vi "Save Object Settings.vi"(8 "error in":errorcluster, 10 "Settings":T5={"Paths"=[refnum, refnum, refnum], "Rectangles"=[refnum, refnum], "Funnels"=[refnum, refnum, refnum, refnum, refnum, refnum], "Dots"=[refnum, refnum, refnum, refnum, refnum, refnum, refnum, refnum, refnum]}, 11 "Archivist in":refnum<class "Archivist.lvclass">) -> (0 "error out":errorcluster, 3 "Archivist out":refnum<class "Archivist.lvclass">)   [LabVIEW 2019, in "Archivist.lvclass"]
uses:
  Archivist.lvclass
  Settings/Setting Database/Typedefs/PublicEvents--Setting Database.PathsUpdated.ctl
  Settings/Path Settings/Path Settings.lvclass
  Settings/Setting Database/Typedefs/PublicEvents--Setting Database.RectanglesUpdated.ctl
  Settings/Rectangle Settings/Rectangle Settings.lvclass
  Settings/Setting Database/Typedefs/PublicEvents--Setting Database.FunnelsUpdated.ctl
  Settings/Funnel Settings/Funnel Settings.lvclass
  Settings/Setting Database/Typedefs/PublicEvents--Setting Database.DotsUpdated.ctl
  Settings/Dot Settings/Dot Settings.lvclass
  Settings/Setting Database/Setting Database.lvclass
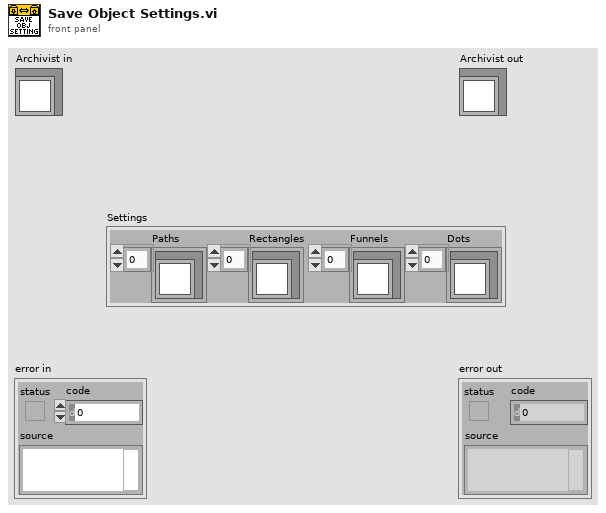
[diagram p1: front panel]
types:
  T1 = typedef "Setting Database.lvclass/PublicEvents--Setting Database.PathsUpdated.ctl" = refnum<class "Path Settings.lvclass">[]
  T2 = typedef "Setting Database.lvclass/PublicEvents--Setting Database.RectanglesUpdated.ctl" = refnum<class "Rectangle Settings.lvclass">[]
  T3 = typedef "Setting Database.lvclass/PublicEvents--Setting Database.FunnelsUpdated.ctl" = refnum<class "Funnel Settings.lvclass">[]
  T4 = typedef "Setting Database.lvclass/PublicEvents--Setting Database.DotsUpdated.ctl" = refnum<class "Dot Settings.lvclass">[]
  T5 = cluster{"Paths":T1, "Rectangles":T2, "Funnels":T3, "Dots":T4}
  T6 = enum16{"open", "replace", "create", "open or create", "replace or create", "replace or create with confirmation"}
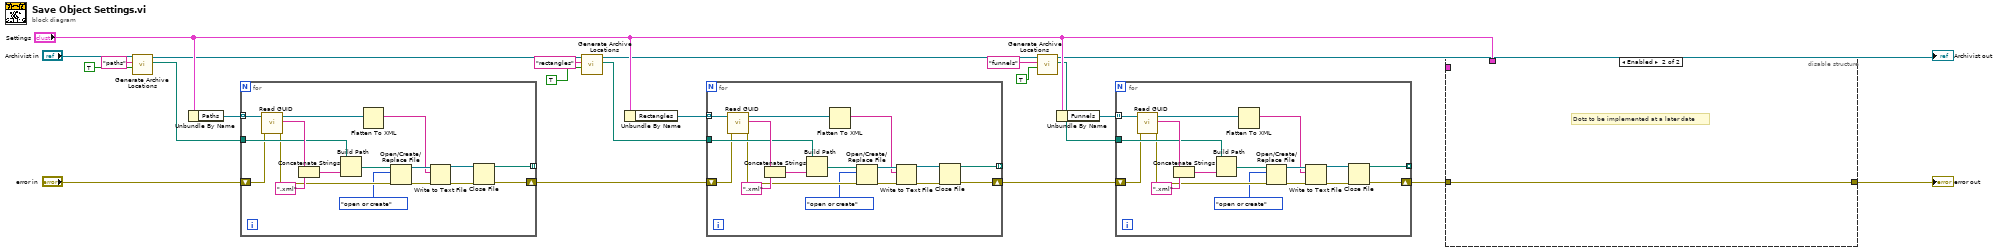
[diagram p0: block diagram]
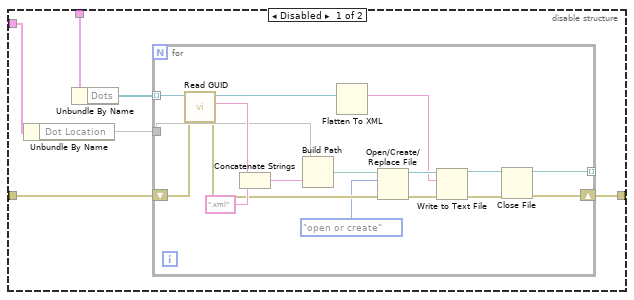
[diagram p2: hidden frame]
diagram:
  n1 = call "Generate Archive Locations.vi"("Archive?"=TRUE, "Key"="paths", "Archivist In"="Archivist in") -> ("Path Out"=w13:path, "Archivist Out"=w10:refnum<class "Archivist.lvclass">)  [unwired: 7 in]
  n2 = Unbundle By Name("Settings") -> ("Paths"=w21:T1)
  n3 = for {
    tunnel: w13 -> [w36]
    tunnel: w21 -> [w39] mode=indexing
    tunnel: [w27] -> _ mode=indexing
    shift-right: [w26] -> w3
    shift-left: "error in" -> [w25]
    n4 = call-dynamic "Read GUID.vi"("error in (no error)"=w25, "ObjectSettings in"=w39) -> ("error out"=w30:errorcluster, "GUID"=w37:string, "ObjectSettings out"=w34:refnum<class "Path Settings.lvclass">)  [unwired: 7 in]
    n5 = Concatenate Strings(w37, ".xml" ("string")) -> (w35:string)
    n6 = Build Path(base path=w36, name or relative path=w35) -> (appended path=w33:path)
    n7 = Flatten To XML(anything=w34) -> (xml string=w24:string)
    n8 = Open/Create/Replace File(file path (use dialog)=w33, error in=w30, operation (0:open)=T6."open or create") -> (refnum out=w32:refnum<file>, error out=w31:errorcluster)  [unwired: 3 in, 1 out]
    n9 = Write to Text File(file (use dialog)=w32, text=w24, error in=w31) -> (refnum out=w28:refnum<file>, error out=w29:errorcluster)  [unwired: 1 in, 1 out]
    n10 = Close File(refnum=w28, error in=w29) -> (path=w27:path, error out=w26:errorcluster)
  }
  n11 = call "Generate Archive Locations.vi"("Archive?"=TRUE, "Key"="rectangles", "Archivist In"=w10) -> ("Path Out"=w9:path, "Archivist Out"=w7:refnum<class "Archivist.lvclass">)  [unwired: 7 in]
  n12 = Unbundle By Name("Settings") -> ("Rectangles"=w20:T2)
  n13 = for {
    tunnel: w9 -> [w53]
    tunnel: w20 -> [w56] mode=indexing
    tunnel: [w44] -> _ mode=indexing
    shift-right: [w43] -> w2
    shift-left: w3 -> [w42]
    n14 = call-dynamic "Read GUID.vi"("error in (no error)"=w42, "ObjectSettings in"=w56) -> ("error out"=w47:errorcluster, "GUID"=w54:string, "ObjectSettings out"=w51:refnum<class "Rectangle Settings.lvclass">)  [unwired: 7 in]
    n15 = Concatenate Strings(w54, ".xml" ("string")) -> (w52:string)
    n16 = Build Path(base path=w53, name or relative path=w52) -> (appended path=w50:path)
    n17 = Flatten To XML(anything=w51) -> (xml string=w41:string)
    n18 = Open/Create/Replace File(file path (use dialog)=w50, error in=w47, operation (0:open)=T6."open or create") -> (refnum out=w49:refnum<file>, error out=w48:errorcluster)  [unwired: 3 in, 1 out]
    n19 = Write to Text File(file (use dialog)=w49, text=w41, error in=w48) -> (refnum out=w45:refnum<file>, error out=w46:errorcluster)  [unwired: 1 in, 1 out]
    n20 = Close File(refnum=w45, error in=w46) -> (path=w44:path, error out=w43:errorcluster)
  }
  n21 = call "Generate Archive Locations.vi"("Archive?"=TRUE, "Key"="funnels", "Archivist In"=w7) -> ("Path Out"=w5:path, "Archivist Out"=→"Archivist out":refnum<class "Archivist.lvclass">)  [unwired: 7 in]
  n22 = Unbundle By Name("Settings") -> ("Funnels"=w19:T3)
  n23 = for {
    tunnel: w5 -> [w70]
    tunnel: w19 -> [w73] mode=indexing
    tunnel: [w61] -> _ mode=indexing
    shift-right: [w60] -> w18
    shift-left: w2 -> [w59]
    n24 = call-dynamic "Read GUID.vi"("error in (no error)"=w59, "ObjectSettings in"=w73) -> ("error out"=w64:errorcluster, "GUID"=w71:string, "ObjectSettings out"=w68:refnum<class "Funnel Settings.lvclass">)  [unwired: 7 in]
    n25 = Concatenate Strings(w71, ".xml" ("string")) -> (w69:string)
    n26 = Build Path(base path=w70, name or relative path=w69) -> (appended path=w67:path)
    n27 = Flatten To XML(anything=w68) -> (xml string=w58:string)
    n28 = Open/Create/Replace File(file path (use dialog)=w67, error in=w64, operation (0:open)=T6."open or create") -> (refnum out=w66:refnum<file>, error out=w65:errorcluster)  [unwired: 3 in, 1 out]
    n29 = Write to Text File(file (use dialog)=w66, text=w58, error in=w65) -> (refnum out=w62:refnum<file>, error out=w63:errorcluster)  [unwired: 1 in, 1 out]
    n30 = Close File(refnum=w62, error in=w63) -> (path=w61:path, error out=w60:errorcluster)
  }
  n31 = disable-structure shown="Enabled" {
    disable-tunnel: w18 -> [w77 w97]
    disable-tunnel: _ -> [w76 _]
    disable-tunnel: "Settings" -> [w75 _]
    disable-tunnel: [w74 w97] -> w16
    frame Disabled {
      n32 = Unbundle By Name(w76) -> ("Dot Location"=w78)
      n33 = Unbundle By Name(w75) -> ("Dots"=w79:T4)
      n34 = for {
        tunnel: w78 -> [w93]
        tunnel: w79 -> [w96] mode=indexing
        tunnel: [w84] -> _ mode=indexing
        shift-right: [w83] -> w74
        shift-left: w77 -> [w82]
        n35 = call-dynamic "Read GUID.vi"("error in (no error)"=w82, "ObjectSettings in"=w96) -> ("error out"=w87:errorcluster, "GUID"=w94:string, "ObjectSettings out"=w91:refnum<class "Dot Settings.lvclass">)  [unwired: 7 in]
        n36 = Concatenate Strings(w94, ".xml" ("string")) -> (w92:string)
        n37 = Build Path(base path=w93, name or relative path=w92) -> (appended path=w90:path)
        n38 = Flatten To XML(anything=w91) -> (xml string=w81:string)
        n39 = Open/Create/Replace File(file path (use dialog)=w90, error in=w87, operation (0:open)=T6."open or create") -> (refnum out=w89:refnum<file>, error out=w88:errorcluster)  [unwired: 3 in, 1 out]
        n40 = Write to Text File(file (use dialog)=w89, text=w81, error in=w88) -> (refnum out=w85:refnum<file>, error out=w86:errorcluster)  [unwired: 1 in, 1 out]
        n41 = Close File(refnum=w85, error in=w86) -> (path=w84:path, error out=w83:errorcluster)
      }
    }
    frame Enabled {
      # "Dots to be implemented at a later date"
    }
  }
  "error out" <- w16
